vi "FEMC_Get_Rev_Level.vi"(4 "error in":errorcluster {"code" format="%.0x"}, 5 "Slave Node in":cluster{"Address":i8, "Serial Number":i8[]} {"Serial Number" format="%.0x"; "Address" format="%.0x"}, 6 "RCA":u32=196608 format="%x", 7 "ObjHandle in":u32) -> (0 "error out":errorcluster {"code" format="%.0x"}, 1 "Revision Level out":string, 3 "ObjHandle out":u32)   [LabVIEW 2017]
doc: "Request the revision level of the code in a slave node.\nThe revision level is returned as a string in the format Vw.x.y.z"
panel:
  # "ALMA Monitor and Control Bus\nGet FEMC Revision Level"
  # "Node Address"
  # "Serial Number"
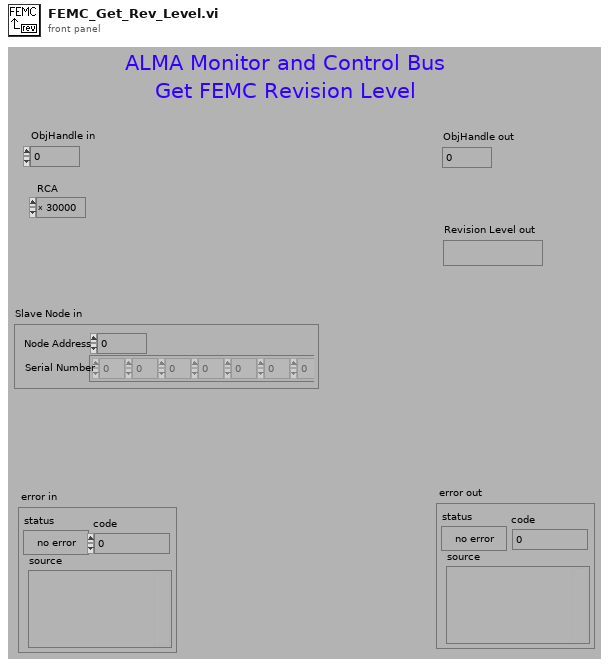
[diagram p1: front panel]
types:
  T1 = cluster{"Data Array out[0]":u8, "Data Array out[1]":u8, "Data Array out[2]":u8}
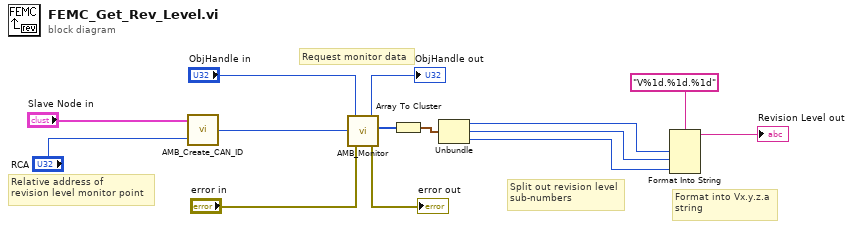
[diagram p0: block diagram]
diagram:
  # "Format into Vx.y.z.a\nstring"
  # "Split out revision level\nsub-numbers"
  # "Request monitor data"
  # "Relative address of\nrevision level monitor point"
  n1 = call "AMB_Create_CAN_ID.vi"("Relative Address in"="RCA", "Slave Node in"="Slave Node in") -> ("CAN ID out"=w12:u32)
  n2 = call "AMB_Monitor.vi"("ObjHandle in"="ObjHandle in", "CAN ID in"=w12, "error in"="error in") -> ("ObjHandle out"=→"ObjHandle out":u32, "Data Array out"=w6:u8[], "error out"=→"error out":errorcluster)  [unwired: 1 out]
  n3 = Array To Cluster(array=w6) -> (cluster=w5:T1)
  n4 = Unbundle(w5) -> ("Data Array out[0]"=w3:u8, "Data Array out[1]"=w2:u8, "Data Array out[2]"=w1:u8)
  n5 = Format Into String(format string="V%1d.%1d.%1d" ("Format String"), w3, w2, w1) -> (resulting string=→"Revision Level out":string)  [unwired: 2 in, 1 out]
